vi "CPP_Aeroprobe_dT-Unified.vi"() -> (5 "Plug in titles":string[](array[string]), 7 "Plug in values":string[](array[string]))   [LabVIEW 2013]
uses:
  Plug in sub vis/CPP_Aeroprobe/SanityCluster.ctl
  <vilib>/Analysis/baseanly.llb/Mean (DBL).vi
  Globals/Meas_global.vi
  Globals/Trav_pos_global.vi
  <vilib>/Analysis/NI_AALBase.lvlib
panel:
  in  "Mode":enum32{"Measure", "Take Zeroes"}(radio)
  in  "RunManually?":bool
  in  "MeanOrFull":bool
  in  "Graphs":bool
  in  "Downsampler":i32=80
  in  "Calibration Folder Path":path=path "M:/Preferences/Rig_Setups/All_Rigs/Calibrations/5HoleProbeRegrid"
  in  "Correction File Path":path=path "M:/Preferences/Rig_Setups/All_Rigs/TubingCompensation/5HPTubingCorrection12066.xls"
  # "!! 5-hole 1-5 must be connected to Channels 1-5 !!"
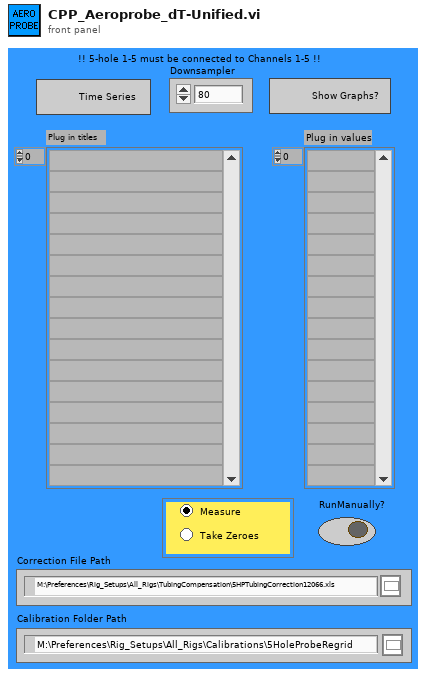
[diagram p1: front panel]
types:
  T1 = typedef "SanityCluster.ctl" = cluster{"PressureErrors":bool[][], "Plug in titles":string[]}
  T2 = typedef "Post_Process.ctl" = enum16{"Take New Data", "Post Process Raw Data File"}
  T3 = typedef "Traverse_cluster.ctl" = cluster{"Start X":dbl, "Start Y":dbl, "Start Z":dbl, "End X":dbl, "End Y":dbl, "End Z":dbl, "No. of pts.":i32, "Spacing":T4, "Filename":path, "Tunnel Speed":dbl, "Averaging time (min)":dbl, "Extra Commands":string, "Specific Arguments":string, "Emission Rate (l/min)":dbl, "Trace Gas Concentration (%)":dbl, "Density Ratio":string, "Comments":string, "Row No":i32, "Row Type Selector":T5, "Completion time":string, "Row Duration (mins)":dbl, "No. of Valid pts.":i32, "Meas Setup File":string}
  T4 = typedef "Spacing.ctl" = enum16{"Linear", "Log", "Gauss", "Specified", "N/A"}
  T5 = typedef "Multi_run_mode.ctl" = enum16{"Move Traverse Only", "Set Tunnel Speed Only", "Set Source Only", "Set Measurement Conditions", "Single Measurement", "Vertical Profile", "Lateral Profile", "Longitudinal Profile", "Explore Volume", "Multi-Axis Profile", "Auto Calibrate", "Meas Fast FID Bkgnd", "Check Beam Power", "Scanning Valve Measurement", "Run VI Named:", "Set ADAM Ch", "Wait (minutes)", "Send Message", "Synchronize With:", "Fall Back to this Row", "Turn Off Row Repeating", "Blank Row", "Traverse 3D Volume"}
  T6 = typedef "Analysis_info_cluster.ctl" = cluster{"Colour":u32, "Inst type":T7, "Inst name":string, "Symbol":string, "Code name":string, "Extra Info":string, "Inst Array":T8, "Extra Titles":string[], "Extra Values":string[], "U":dbl, "u^2":dbl, "u^3":dbl, "u^4":dbl, "Skew_u":dbl, "Kurt_u":dbl, "Sd Error in Mean":dbl, "% u'/U":dbl, "X":dbl, "Y":dbl, "Z":dbl, "Timescale integral to 25%":dbl, "Sd Error in Variance":dbl, "Calib File":path, "Calib Constants":dbl[], "Output Position":bool, "Full Stats":bool, "Av Sampling Rate":dbl, "Av No of Samples":dbl, "Total Meas Time (s)":dbl, "ADAM Ch Name":string}
  T7 = typedef "Inst_type.ctl" = enum16{"Propeller anemometer", "Raw voltage", "Pressure Transducer", "Pitot-static tube", "Preston tube", "Hot wire", "Cross wire 1", "Cross wire 2", "Generic Linear", "Generic Polynomial", "Generic BackPoly", "Fast FID", "Thermocouple", "Cold wire", "Pulsed Wire", "LDA Vel", "LDA Tran time", "LDA Arr time"}
  T8 = typedef "Instrument_Array.ctl" = enum16{"PWA", "LDA", "Analogue"}
  T9 = cluster{"Analysis Info cluster[0]":T6, "Analysis Info cluster[1]":T6, "Analysis Info cluster[2]":T6, "Analysis Info cluster[3]":T6, "Analysis Info cluster[4]":T6, "Analysis Info cluster[5]":T6, "Analysis Info cluster[6]":T6}
  T10 = typedef "Time_Trace_Cluster.ctl" = cluster{"Weighting":dbl[], "Time (s)":dbl[], "Voltage":dbl[], "Eng Values":dbl[]}
  T11 = typedef "GoodArray.ctl" = bool[]
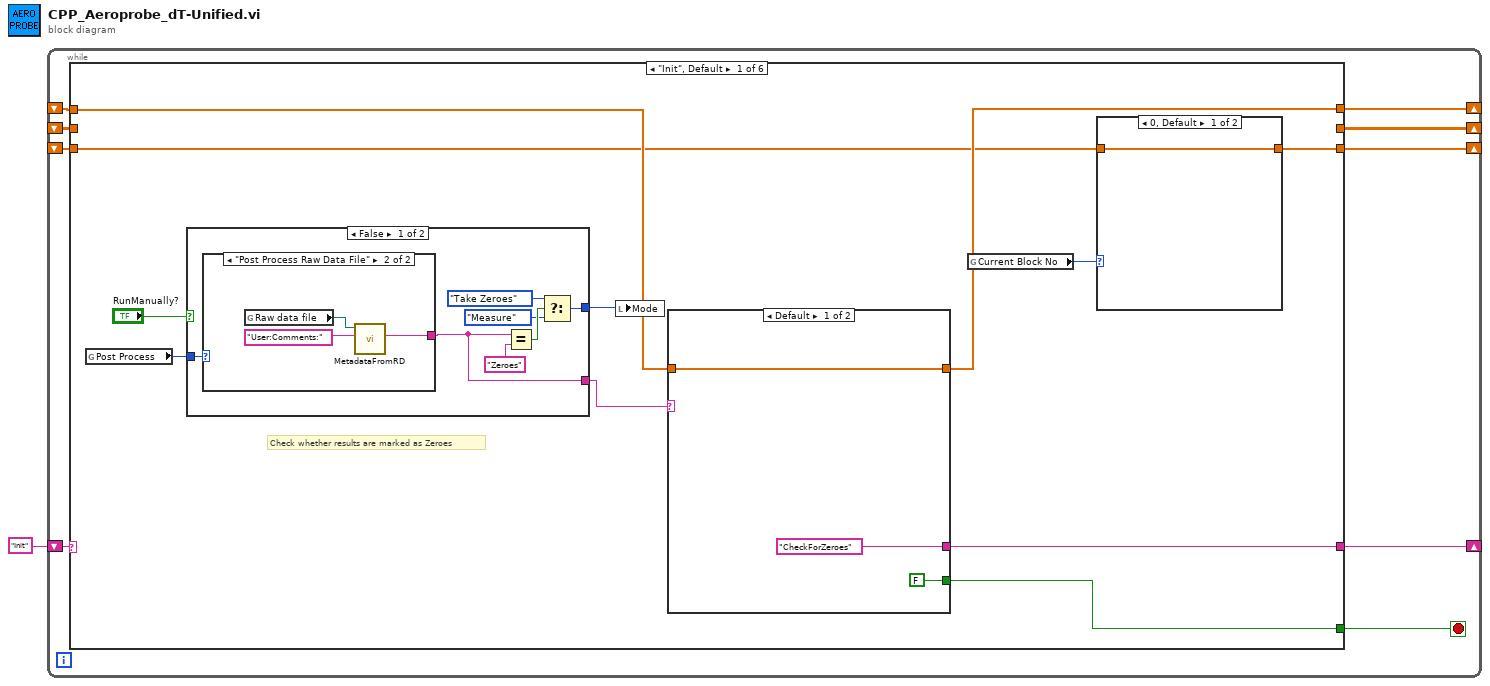
[diagram p0: block diagram]
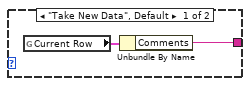
[diagram p2: hidden frame]
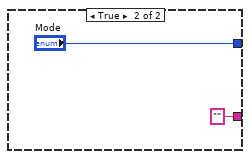
[diagram p3: hidden frame]
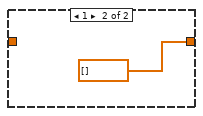
[diagram p4: hidden frame]
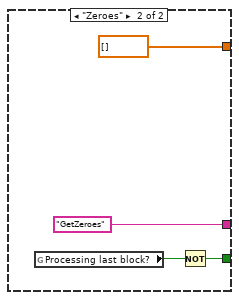
[diagram p5: hidden frame]
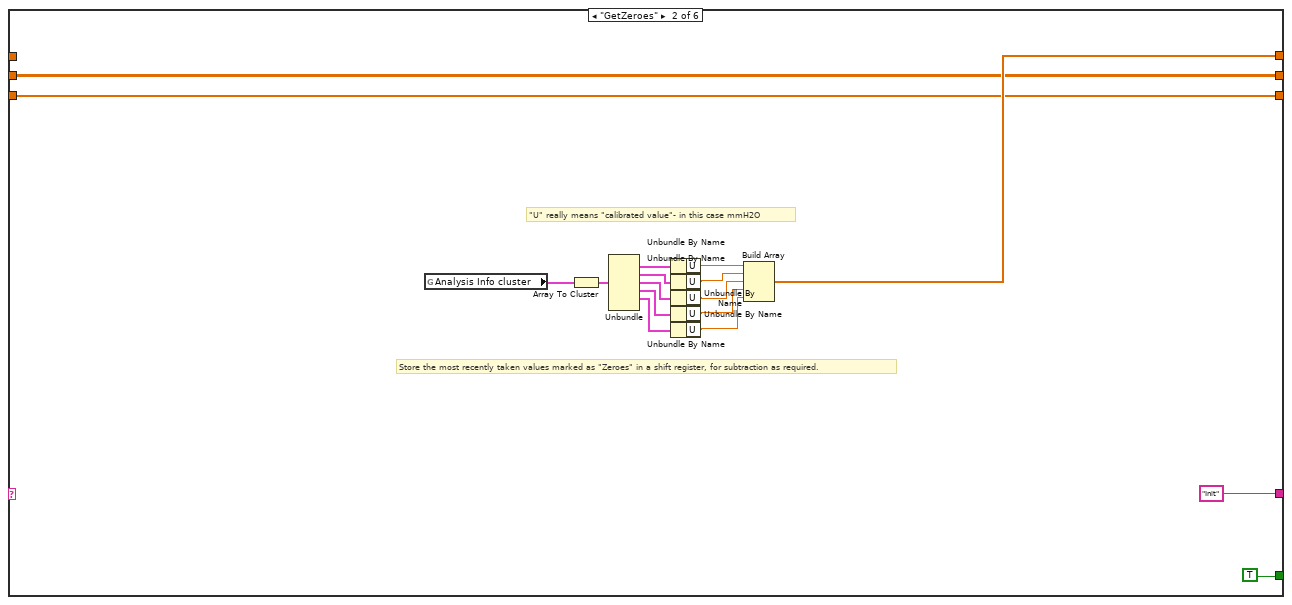
[diagram p6: hidden frame]
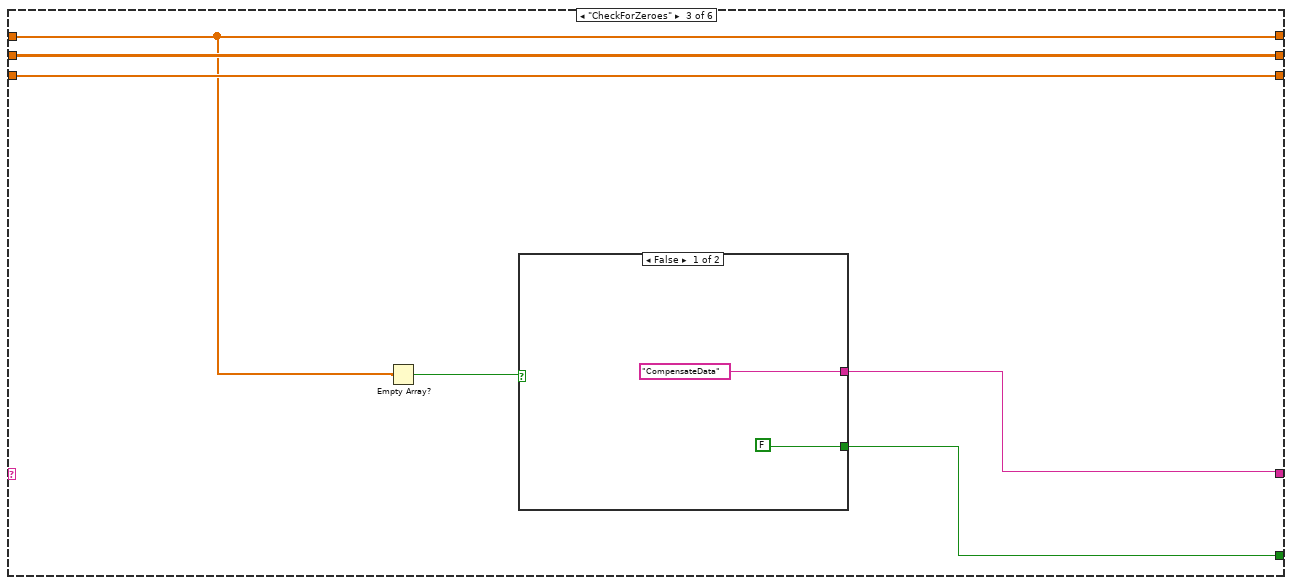
[diagram p7: hidden frame]
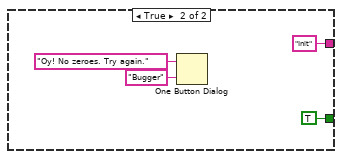
[diagram p8: hidden frame]
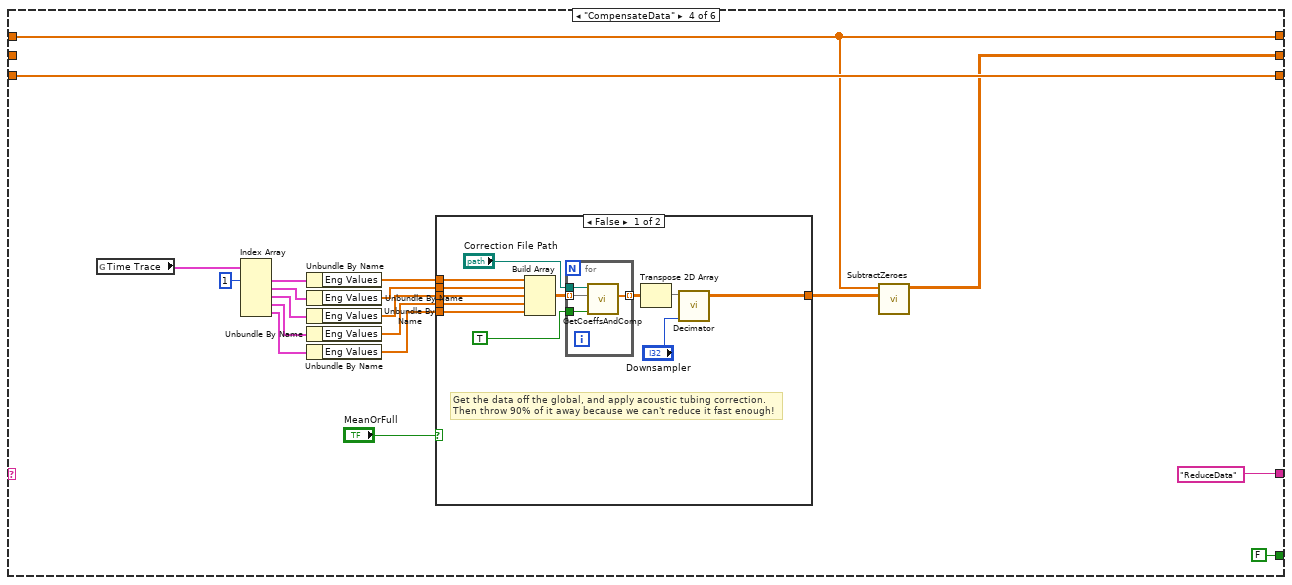
[diagram p9: hidden frame]
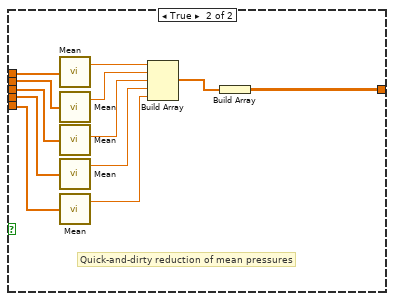
[diagram p10: hidden frame]
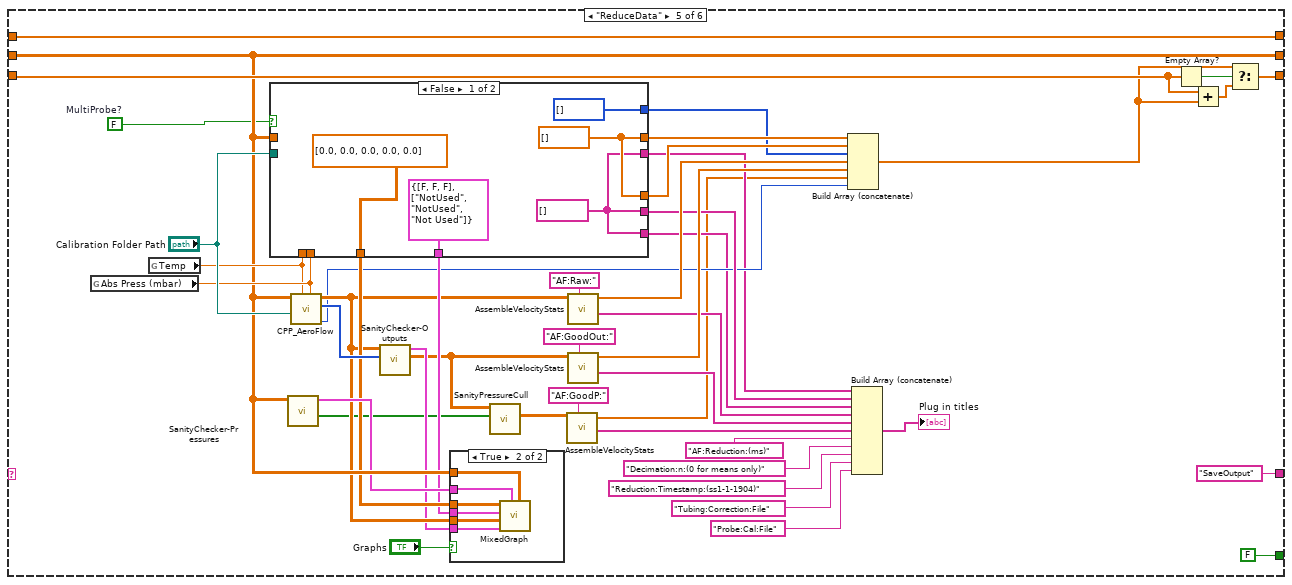
[diagram p11: hidden frame]
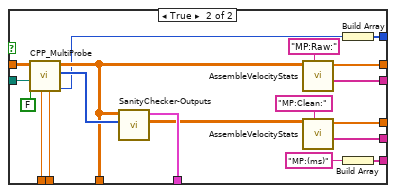
[diagram p12: hidden frame]
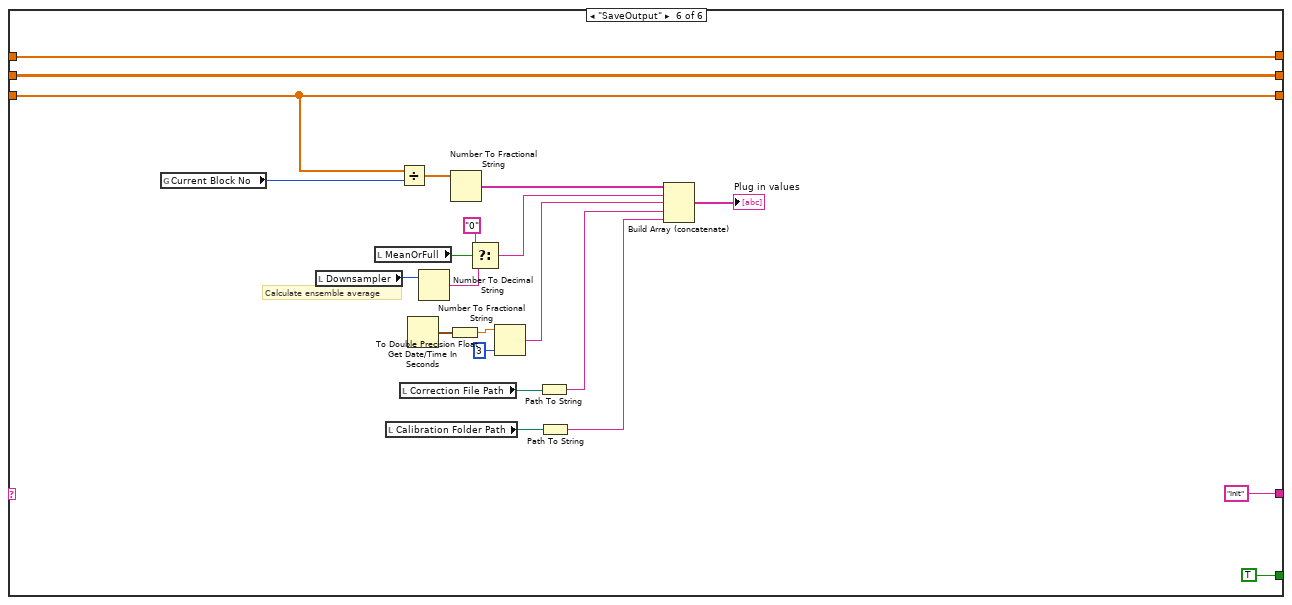
[diagram p14: hidden frame]
diagram:
  n1 = while {
    shift-right: [w9] -> _
    shift-left: "Init" -> [w10]
    shift-right: [w8] -> _
    shift-left: _ -> [w7]
    shift-right: [w6] -> _
    shift-left: _ -> [w5]
    shift-right: [w3] -> _
    shift-left: _ -> [w2]
    stop <- w4 stop-if-true
    n2 = case shown="\"Init\", Default" w10 {
      tunnel: [w21 "Init" w66 "ReduceData" "SaveOutput" "Init"] -> w9
      tunnel: [w18 w48 w63 w78 w164 w217] -> w8
      tunnel: w7 -> [w19 _ w63 w78 w164 w217]
      tunnel: [w17 w46 w67 w92 w159 w211] -> w6
      tunnel: w5 -> [w16 w46 w67 w92 w162 w211]
      tunnel: [w20 TRUE w65 FALSE FALSE TRUE] -> w4
      tunnel: [_ w45 w64 w75 w151 w213] -> w3
      tunnel: w2 -> [_ w45 w64 _ w151 w213]
      frame "Init", Default {
        # "Check whether results are marked as Zeroes"
        n3 = global read "Meas_global.vi" "Post Process"() -> (w12:T2)
        n4 = case shown="False" "RunManually?" {
          tunnel: [w28 "Mode"] -> w13
          tunnel: w12 -> [w23 _]
          tunnel: [w22 "" ("ValueString")] -> w11
          frame False {
            n5 = case shown="\"Post Process Raw Data File\"" w23 {
              tunnel: [w29 w31] -> w22
              frame "Take New Data", Default {
                n6 = global read "Trav_pos_global.vi" "Current Row"() -> (w30:T3)
                n7 = Unbundle By Name(w30) -> ("Comments"=w29:string)
              }
              frame "Post Process Raw Data File" {
                n8 = global read "Meas_global.vi" "Raw data file"() -> (w33:path)
                n9 = call "MetadataFromRD.vi"("ChannelName"="User:Comments:", "Raw data file"=w33) -> ("ValueString"=w31:string)  [unwired: 8 in, 1 out]
              }
            }
            n10 = Equal?(x=w22, y="Zeroes") -> (x = y?=w26:bool)
            n11 = Select(t=enum32{"Measure", "Take Zeroes"}."Take Zeroes" ("Mode"), s=w26, f=enum32{"Measure", "Take Zeroes"}."Measure" ("Mode")) -> (s? t:f=w28:enum32{"Measure", "Take Zeroes"})
          }
          frame True {
          }
        }
        n12 = local write "Mode"(w13) -> ()
        n13 = case shown="Default" w11 {
          tunnel: ["CheckForZeroes" "GetZeroes"] -> w21
          tunnel: [FALSE w43] -> w20
          tunnel: w19 -> [w38 _]
          tunnel: [w38 dbl[] [] ("t")] -> w18
          frame Default {
          }
          frame "Zeroes" {
            n14 = global read "Meas_global.vi" "Processing last block?"() -> (w42:bool)
            n15 = Not(x=w42) -> (.not. x?=w43:bool)
          }
        }
        n16 = global read "Meas_global.vi" "Current Block No"() -> (w15:i32)
        n17 = case shown="0, Default" w15 {
          tunnel: [w36 dbl[] [] ("t")] -> w17
          tunnel: w16 -> [w36 _]
          frame 0, Default {
          }
          frame 1 {
          }
        }
      }
      frame "GetZeroes" {
        # "Store the most recently taken values marked as \"Zeroes\" in a shift register, for subtraction as required."
        # "\"U\" really means \"calibrated value\"- in this case mmH2O"
        n18 = global read "Meas_global.vi" "Analysis Info cluster"() -> (w50:T6[])
        n19 = Array To Cluster(array=w50) -> (cluster=w56:T9)
        n20 = Unbundle(w56) -> ("Analysis Info cluster[1]"=w57:T6, "Analysis Info cluster[2]"=w58:T6, "Analysis Info cluster[3]"=w59:T6, "Analysis Info cluster[4]"=w60:T6, "Analysis Info cluster[5]"=w61:T6)  [unwired: 2 out]
        n21 = Unbundle By Name(w57) -> ("U"=w55:dbl)
        n22 = Unbundle By Name(w58) -> ("U"=w54:dbl)
        n23 = Unbundle By Name(w59) -> ("U"=w53:dbl)
        n24 = Unbundle By Name(w60) -> ("U"=w52:dbl)
        n25 = Unbundle By Name(w61) -> ("U"=w51:dbl)
        n26 = Build Array(w55, w54, w53, w52, w51) -> (w48:dbl[])
      }
      frame "CheckForZeroes" {
        n27 = Empty Array?(array=w63) -> (empty?=w62:bool)
        n28 = case shown="False" w62 {
          tunnel: ["CompensateData" "Init"] -> w66
          tunnel: [FALSE TRUE] -> w65
          frame False {
          }
          frame True {
            n29 = One Button Dialog(message="Oy! No zeroes. Try again.", button name ("OK")="Bugger") -> ()  [unwired: 1 out]
          }
        }
      }
      frame "CompensateData" {
        n30 = global read "Meas_global.vi" "Time Trace"() -> (w82:T10[])
        n31 = Index Array(array=w82, index #1=1 ("index")) -> (element #1=w81:T10, element #2=w90:T10, element #3=w89:T10, element #4=w88:T10, element #5=w87:T10)  [unwired: 4 in]
        n32 = Unbundle By Name(w81) -> ("Eng Values"=w80:dbl[])
        n33 = Unbundle By Name(w90) -> ("Eng Values"=w86:dbl[])
        n34 = Unbundle By Name(w89) -> ("Eng Values"=w85:dbl[])
        n35 = Unbundle By Name(w88) -> ("Eng Values"=w84:dbl[])
        n36 = Unbundle By Name(w87) -> ("Eng Values"=w83:dbl[])
        n37 = case shown="False" "MeanOrFull" {
          tunnel: w86 -> [w104 w119]
          tunnel: w85 -> [w103 w118]
          tunnel: w84 -> [w102 w117]
          tunnel: w83 -> [w101 w116]
          tunnel: w80 -> [w100 w120]
          tunnel: [w93 w109] -> w79
          frame False {
            # "Get the data off the global, and apply acoustic tubing correction. \nThen throw 90% of it away because we can't reduce it fast enough!"
            n38 = Build Array(w100, w104, w103, w102, w101) -> (w99:dbl[][])
            n39 = for {
              tunnel: w99 -> [w108] mode=indexing
              tunnel: [w107] -> w96 mode=indexing
              tunnel: TRUE ("Apply Phase Correction?") -> [w106]
              tunnel: "Correction File Path" -> [w105]
              n40 = call "GetCoeffsAndComp.vi"("Apply Phase Correction?"=w106, "mutedData"=w108, "TubingCorrectionFile"=w105) -> ("boostedData"=w107:dbl[])  [unwired: 8 in]
            }
            n41 = Transpose 2D Array(2D array=w96) -> (transposed array=w95:dbl[][])
            n42 = call "Decimator.vi"("Decimator"="Downsampler", "Array In"=w95) -> ("DecimatedArrayOut"=w93:dbl[][])  [unwired: 9 in]
          }
          frame True {
            # "Quick-and-dirty reduction of mean pressures"
            n43 = call-poly <vilib>:"Mean.vi"("X"=w120) -> ("mean"=w115:dbl)  [unwired: 1 out]
            n44 = call-poly <vilib>:"Mean.vi"("X"=w119) -> ("mean"=w114:dbl)  [unwired: 1 out]
            n45 = call-poly <vilib>:"Mean.vi"("X"=w118) -> ("mean"=w113:dbl)  [unwired: 1 out]
            n46 = call-poly <vilib>:"Mean.vi"("X"=w117) -> ("mean"=w112:dbl)  [unwired: 1 out]
            n47 = call-poly <vilib>:"Mean.vi"("X"=w116) -> ("mean"=w111:dbl)  [unwired: 1 out]
            n48 = Build Array(w115, w114, w113, w112, w111) -> (w110:dbl[])
            n49 = Build Array(w110) -> (w109:dbl[][])
          }
        }
        n50 = call "SubtractZeroes.vi"("RawPressure"=w79, "Zeroes"=w78) -> ("ZeroedPressure"=w75:dbl[][])  [unwired: 9 in]
      }
      frame "ReduceData" {
        w132 = FALSE  # MultiProbe?
        n51 = global read "Meas_global.vi" "Abs Press (mbar)"() -> (w156:dbl)
        n52 = global read "Meas_global.vi" "Temp"() -> (w155:dbl)
        n53 = case shown="False" w132 {
          tunnel: [w170 w189] -> w158
          tunnel: "Calibration Folder Path" -> [_ w188]
          tunnel: w156 -> [_ w187]
          tunnel: w155 -> [_ w186]
          tunnel: w151 -> [_ w182]
          tunnel: [dbl[][] [[0.0, 0.0, 0.0, 0.0, 0.0]] ("RawVmagUVWCone") w181] -> w149
          tunnel: [T1 {"PressureErrors"=[[FALSE, FALSE, FALSE]], "Plug in titles"=["NotUsed", "NotUsed", "Not Used"]} ("OutputErrors") w180] -> w148
          tunnel: [w170 w177] -> w143
          tunnel: [w169 w176] -> w140
          tunnel: [u32[] [] w172] -> w135
          tunnel: [w169 w171] -> w134
          tunnel: [w169 w173] -> w133
          frame False {
            w169 = string[] [] ("Plug in titles")
            w170 = dbl[] [] ("StatsArray")
          }
          frame True {
            n54 = call "CPP_MultiProbe.vi"("Pressure (mBar)"=w187, "Temperature (C)"=w186, "Old5HoleProbe?"=FALSE, "Calibration Folder Path"=w188, "ZeroedPressures (mmH2O)"=w182) -> ("Time (ms)"=w175:u32, "ReductionCode"=w183:i32[], "RawVmagUVWCone"=w181:dbl[][])  [unwired: 1 in, 1 out]
            n55 = call "SanityChecker-Outputs.vi"("ReductionCode"=w183, "RawVmagUVWCone"=w181) -> ("SanitisedVmagUVWCone"=w179:dbl[][], "OutputErrors"=w180:T1)  [unwired: 7 in, 1 out]
            n56 = call "AssembleVelocityStats.vi"("TitlePrefix"="MP:Raw:", "VmagUVWCone"=w181) -> ("Plug in titles"=w173:string[], "StatsArray"=w189:dbl[])  [unwired: 8 in]
            n57 = call "AssembleVelocityStats.vi"("TitlePrefix"="MP:Clean:", "VmagUVWCone"=w179) -> ("Plug in titles"=w176:string[], "StatsArray"=w177:dbl[])  [unwired: 8 in]
            n58 = Build Array(w175) -> (w172:u32[])
            n59 = Build Array("MP:(ms)") -> (w171:string[])
          }
        }
        n60 = call "SanityChecker-Pressures.vi"("ZeroedPressures"=w151) -> ("GoodPressures"=w128:T11, "Sanity"=w150:T1)  [unwired: 9 in]
        n61 = call "CPP_AeroFlow.vi"("Pressure (mBar)"=w156, "Temperature (C)"=w155, "Calibration Folder Path"="Calibration Folder Path", "ZeroedPressures (mmH2O)"=w151) -> ("Time(ms)"=w136:u32, "ReductionCode"=w153:i32[], "RawVmagUVWCone"=w147:dbl[][])  [unwired: 2 in, 1 out]
        n62 = call "SanityChecker-Outputs.vi"("ReductionCode"=w153, "RawVmagUVWCone"=w147) -> ("SanitisedVmagUVWCone"=w129:dbl[][], "OutputErrors"=w146:T1)  [unwired: 7 in, 1 out]
        n63 = case shown="True" "Graphs" {
          tunnel: w151 -> [_ w195]
          tunnel: w150 -> [_ w194]
          tunnel: w149 -> [_ w193]
          tunnel: w148 -> [_ w192]
          tunnel: w147 -> [_ w191]
          tunnel: w146 -> [_ w190]
          frame False {
          }
          frame True {
            n64 = call "MixedGraph.vi"("ZeroedPressure"=w195, "PressureSanity"=w194, "OutputErrors2"=w190, "RawVmagUVWCone2"=w191, "OutputErrors1"=w192, "RawVmagUVWCone1"=w193) -> ()  [unwired: 6 in]
          }
        }
        n65 = call "SanityPressureCull.vi"("GoodPressures"=w128, "VmagUVWCone"=w129) -> ("SanitisedVmagUVWCone"=w130:dbl[][])  [unwired: 9 in]
        n66 = call "AssembleVelocityStats.vi"("TitlePrefix"="AF:GoodP:", "VmagUVWCone"=w130) -> ("Plug in titles"=w127:string[], "StatsArray"=w125:dbl[])  [unwired: 8 in]
        n67 = call "AssembleVelocityStats.vi"("TitlePrefix"="AF:Raw:", "VmagUVWCone"=w147) -> ("Plug in titles"=w139:string[], "StatsArray"=w142:dbl[])  [unwired: 8 in]
        n68 = call "AssembleVelocityStats.vi"("TitlePrefix"="AF:GoodOut:", "VmagUVWCone"=w129) -> ("Plug in titles"=w138:string[], "StatsArray"=w141:dbl[])  [unwired: 8 in]
        n69 = Build Array (concatenate)(w158, w143, w135, w142, w141, w125, w136) -> (w144:dbl[])
        n70 = Build Array (concatenate)(w133, w140, w134, w139, w138, w127, "AF:Reduction:(ms)", "Decimation:n:(0 for means only)" ("element"), "Reduction:Timestamp:(ss1-1-1904)" ("element"), "Tubing:Correction:File" ("element"), "Probe:Cal:File" ("element")) -> (→"Plug in titles":string[])
        n71 = Empty Array?(array=w162) -> (empty?=w161:bool)
        n72 = Add(x=w162, y=w144) -> (x+y=w160:dbl[])
        n73 = Select(t=w144, s=w161, f=w160) -> (s? t:f=w159:dbl[])
      }
      frame "SaveOutput" {
        # "Calculate ensemble average"
        n74 = global read "Meas_global.vi" "Current Block No"() -> (w214:i32)
        n75 = local read "Downsampler"() -> (w210:i32)
        n76 = local read "MeanOrFull"() -> (w209:bool)
        n77 = local read "Calibration Folder Path"() -> (w198:path)
        n78 = Divide(x=w211, y=w214) -> (x/y=w212:dbl[])
        n79 = local read "Correction File Path"() -> (w200:path)
        n80 = Get Date/Time In Seconds() -> (seconds since 1Jan1904=w206:timestamp)
        n81 = Number To Decimal String(number=w210) -> (decimal integer string=w208:string)  [unwired: 1 in]
        n82 = To Double Precision Float(number=w206) -> (double precision float=w205:dbl)
        n83 = Number To Fractional String(number=w212) -> (F-format string=w201:string[])  [unwired: 3 in]
        n84 = Select(t="0", s=w209, f=w208) -> (s? t:f=w204:string)
        n85 = Number To Fractional String(number=w205, precision (6)=i16 3) -> (F-format string=w203:string)  [unwired: 2 in]
        n86 = Path To String(path=w200) -> (string=w199:string)
        n87 = Path To String(path=w198) -> (string=w197:string)
        n88 = Build Array (concatenate)(w201, w204, w203, w199, w197) -> (→"Plug in values":string[])
      }
    }
  }
